vi "Get Coincident Pairs.vi"(4 "interp. method":enum16{"nearest", "linear"}(ring)=enum."linear", 6 "Array 2 Time (s) offset (Default 0)":dbl, 8 "Index2":i32, 9 "Index1":i32, 10 "Cluster 2":T2={"Colour"=0, "Inst type"=enum."Pitot-static tube", "Inst name"="Manometer voltage", "Symbol"="U", "Code name"="", "Extra Info"="U", "Inst Array"=enum."PWA", "U"=0.0, "u^2"=0.0, "u^3"=0.0, "u^4"=0.0, "Skew_u"=0.0, "Kurt_u"=0.0, "Sd Error in Mean"=0.0, "% u'/U"=0.0, "X"=0.0, "Y"=0.0, "Z"=0.0, "Timescale integral Estimate"=0.0, "Sd Error in Variance"=0.0, "Calib File"=path "", "Calib Constants"=[], "Output Position"=FALSE, "Stats"=enum."None", "Av Sampling Rate"=0.0, "Av No of Samples"=0.0, "Total Meas Time (s)"=0.0, "OrigChName"="", "Max value"=0.0, "Min value"=0.0, "Req Sample Rate Hz"=0.0, "Sync Delay Time (s)"=0.0, "Ch No"=0, "Device"="", "Use Latest Calib"=FALSE, "Port"="", "Metadata Ch Names"=[], "Metadata Ch Values"=[], "Label"="", "chState"=enum."Solo", "Point Drift"=0.0, "inputConfig"=""} {"Kurt_u" format="%_3g"; "u^4" format="%_3g"; "u^3" format="%_3g"; "Sd Error in Variance" format="%_3g"; "u^2" format="%_3g"; "Sd Error in Mean" format="%_3g"; "U" format="%_3g"; "Sync Delay Time (s)" format="%.4f"; "Total Meas Time (s)" format="%_5g"; "Skew_u" format="%_3g"; "% u'/U" format="%_3g"}, 11 "Cluster 1":T2={"Colour"=0, "Inst type"=enum."Pitot-static tube", "Inst name"="Manometer voltage", "Symbol"="U", "Code name"="", "Extra Info"="U", "Inst Array"=enum."PWA", "U"=0.0, "u^2"=0.0, "u^3"=0.0, "u^4"=0.0, "Skew_u"=0.0, "Kurt_u"=0.0, "Sd Error in Mean"=0.0, "% u'/U"=0.0, "X"=0.0, "Y"=0.0, "Z"=0.0, "Timescale integral Estimate"=0.0, "Sd Error in Variance"=0.0, "Calib File"=path "", "Calib Constants"=[], "Output Position"=FALSE, "Stats"=enum."None", "Av Sampling Rate"=0.0, "Av No of Samples"=0.0, "Total Meas Time (s)"=0.0, "OrigChName"="", "Max value"=0.0, "Min value"=0.0, "Req Sample Rate Hz"=0.0, "Sync Delay Time (s)"=0.0, "Ch No"=0, "Device"="", "Use Latest Calib"=FALSE, "Port"="", "Metadata Ch Names"=[], "Metadata Ch Values"=[], "Label"="", "chState"=enum."Solo", "Point Drift"=0.0, "inputConfig"=""} {"Kurt_u" format="%_3g"; "u^4" format="%_3g"; "u^3" format="%_3g"; "Sd Error in Variance" format="%_3g"; "u^2" format="%_3g"; "Sd Error in Mean" format="%_3g"; "U" format="%_3g"; "Sync Delay Time (s)" format="%.4f"; "Total Meas Time (s)" format="%_5g"; "Skew_u" format="%_3g"; "% u'/U" format="%_3g"}) -> (0 "Pairs":cluster{"Cluster":T1, "Cluster":T1, dbl}, 3 "Need to Update":bool)   [LabVIEW 2022 SP3]
uses:
  Globals/Meas_global.vi
  Controls/Inst_type.ctl
  Controls/Instrument_Array.ctl
  Controls/Analysis_info_cluster.ctl
  Controls/Resample mode.ctl
  Controls/channelState.ctl
panel:
  out "Array":cluster{"Index1":i32, "Index2":i32}[](array[cluster])
  out "Time Window (ms)":dbl
  out "Frame":string
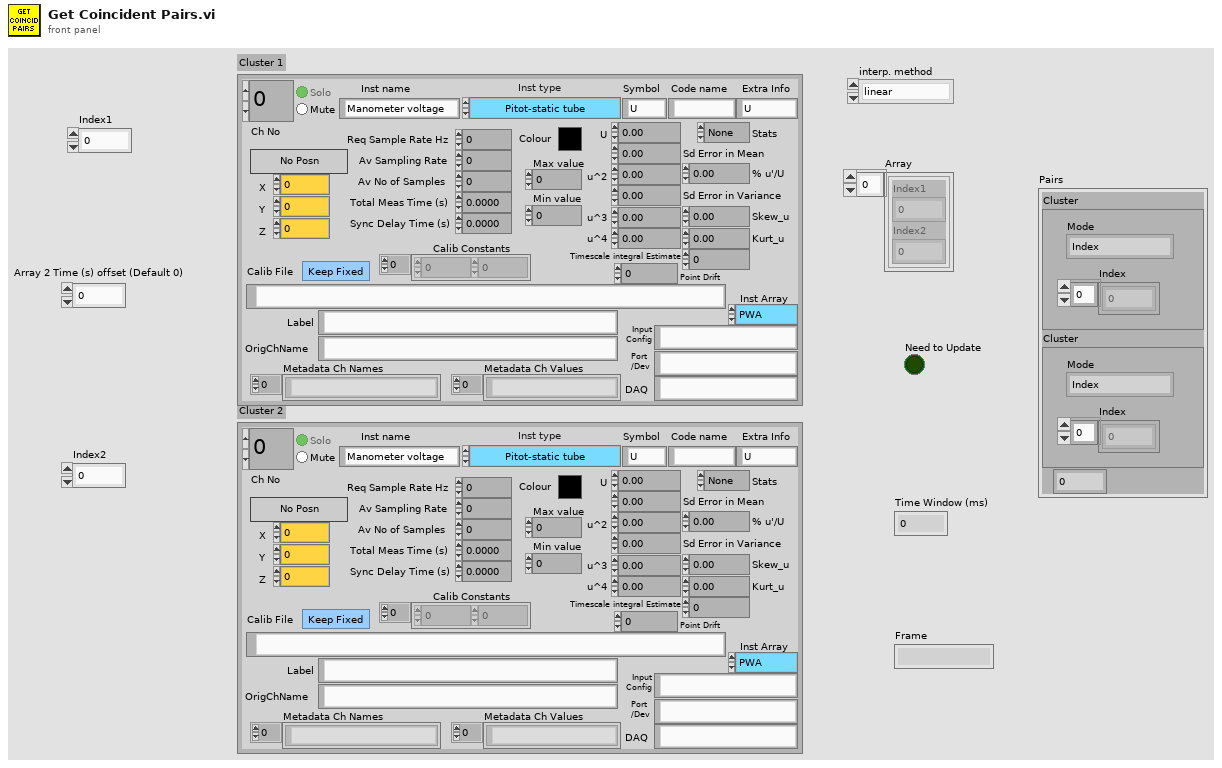
[diagram p1: front panel]
types:
  T1 = typedef "Resample mode.ctl" = cluster{"Mode":enum16{"Index", "Interpolate"}, "Index":dbl[]}
  T2 = typedef "Analysis_info_cluster.ctl" = cluster{"Colour":u32, "Inst type":T3, "Inst name":string, "Symbol":string, "Code name":string, "Extra Info":string, "Inst Array":T4, "U":dbl, "u^2":dbl, "u^3":dbl, "u^4":dbl, "Skew_u":dbl, "Kurt_u":dbl, "Sd Error in Mean":dbl, "% u'/U":dbl, "X":dbl, "Y":dbl, "Z":dbl, "Timescale integral Estimate":dbl, "Sd Error in Variance":dbl, "Calib File":path, "Calib Constants":dbl[], "Output Position":bool, "Stats":enum16{"None", "Basic", "Full"}, "Av Sampling Rate":dbl, "Av No of Samples":dbl, "Total Meas Time (s)":dbl, "OrigChName":string, "Max value":dbl, "Min value":dbl, "Req Sample Rate Hz":dbl, "Sync Delay Time (s)":dbl, "Ch No":i16, "Device":string, "Use Latest Calib":bool, "Port":string, "Metadata Ch Names":string[], "Metadata Ch Values":string[], "Label":string, "chState":T5, "Point Drift":dbl, "inputConfig":string}
  T3 = typedef "Inst_type.ctl" = enum16{"Raw voltage", "Raw with zero offsetting", "Propeller anemometer", "Pressure Transducer", "Pitot-static tube", "Hot wire", "Cross wire 1", "Cross wire 2", "Generic Linear", "Generic Polynomial", "Generic BackPoly", "Fast FID", "Thermocouple", "Cold wire", "Pulsed Wire", "LDA Vel", "LDA Tran time", "LDA Arr time", "Microphone"}
  T4 = typedef "Instrument_Array.ctl" = enum16{"PWA", "LDA", "Analogue"}
  T5 = typedef "channelState.ctl" = enum32{"No Selection", "Solo", "Mute"}
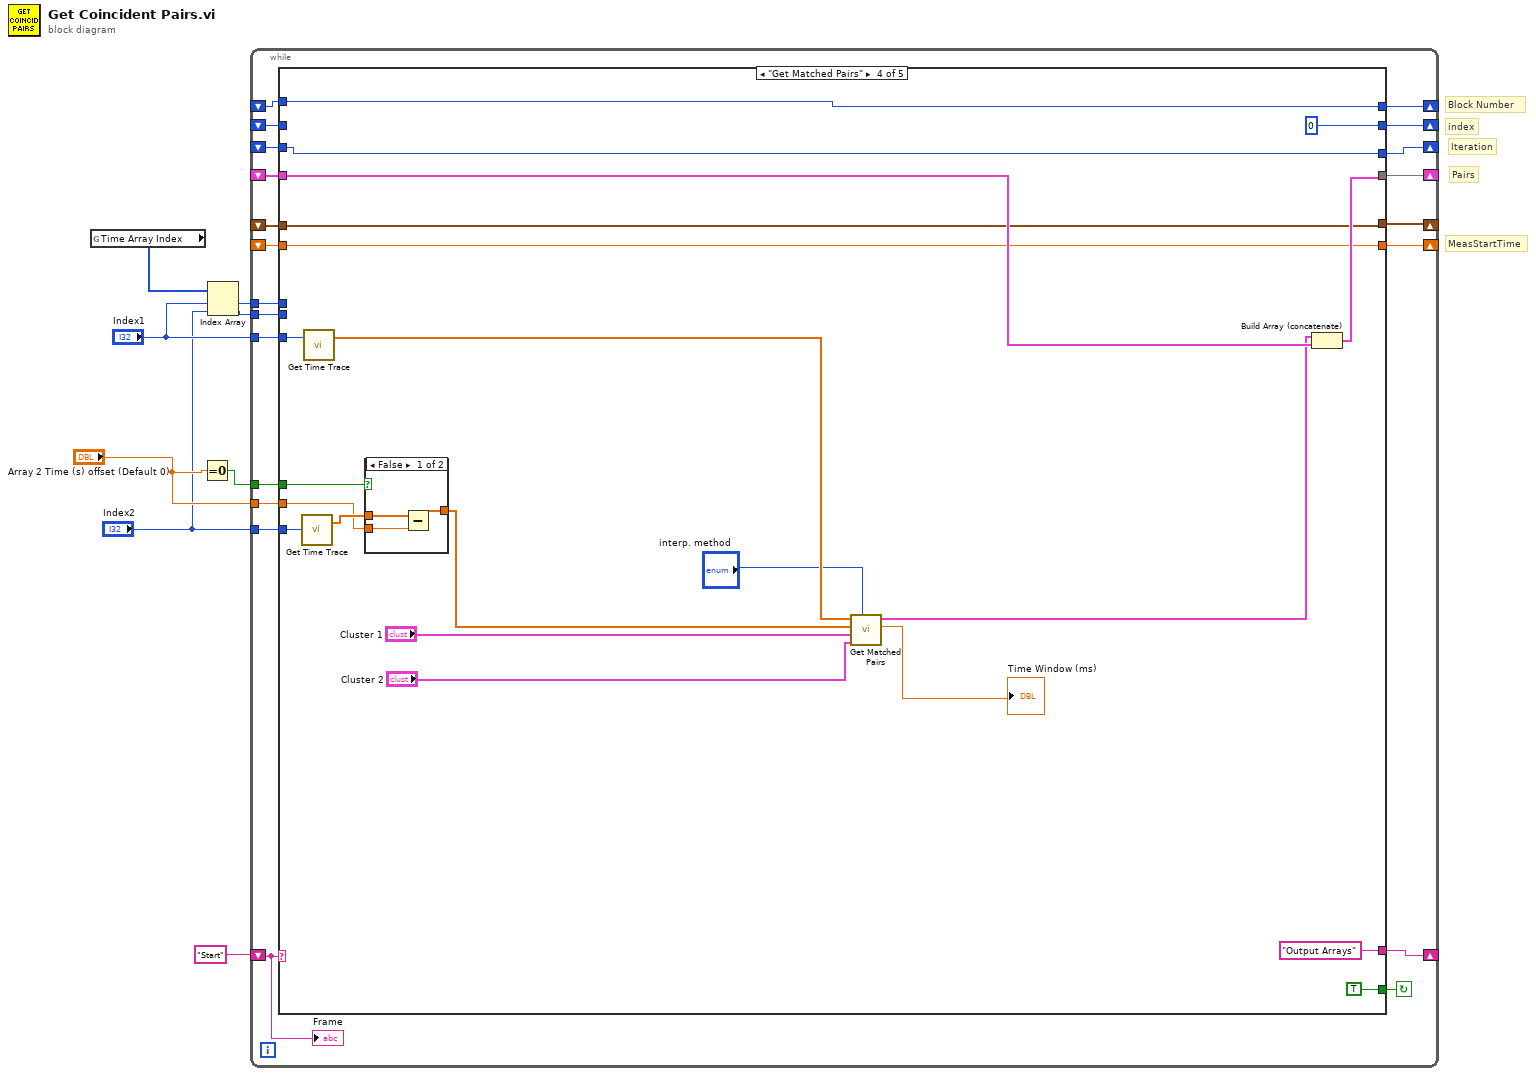
[diagram p0: block diagram]
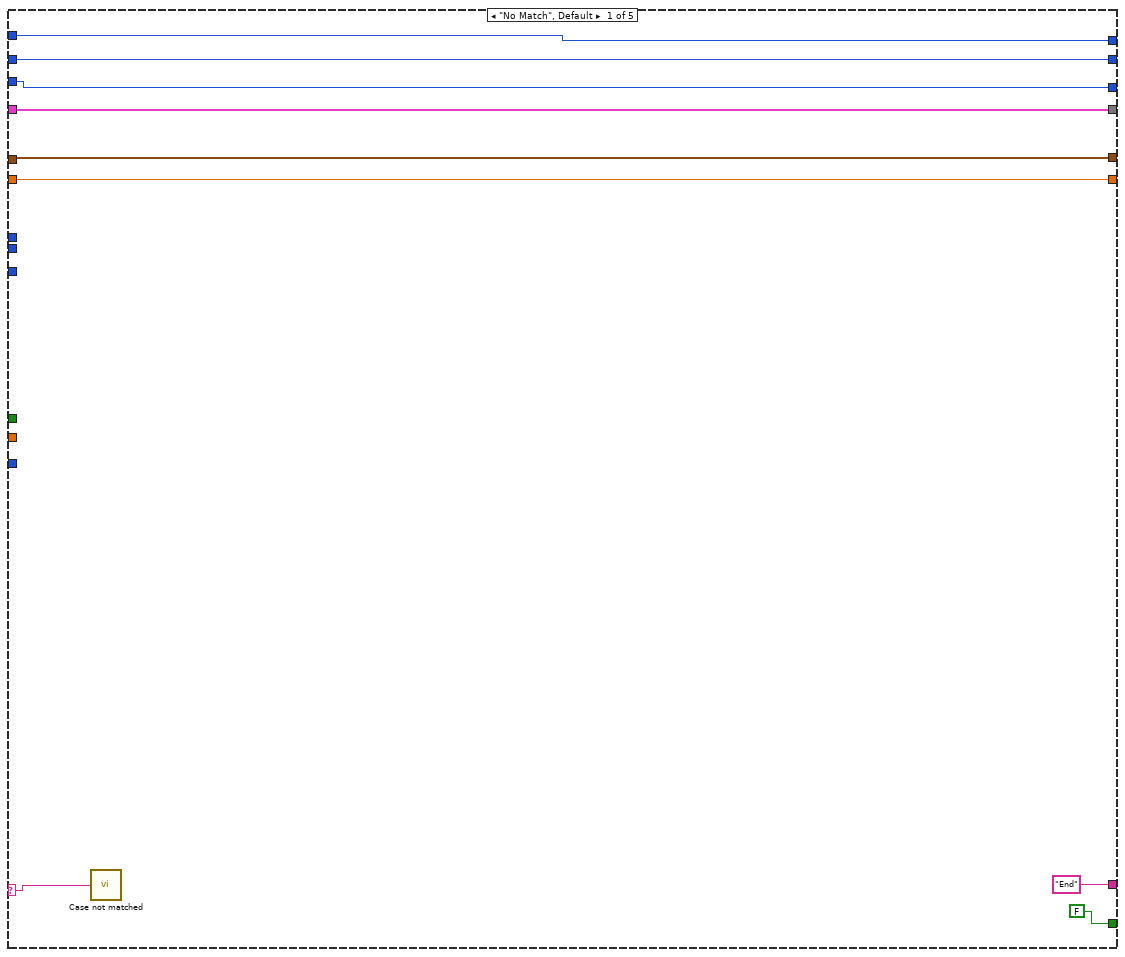
[diagram p2: hidden frame]
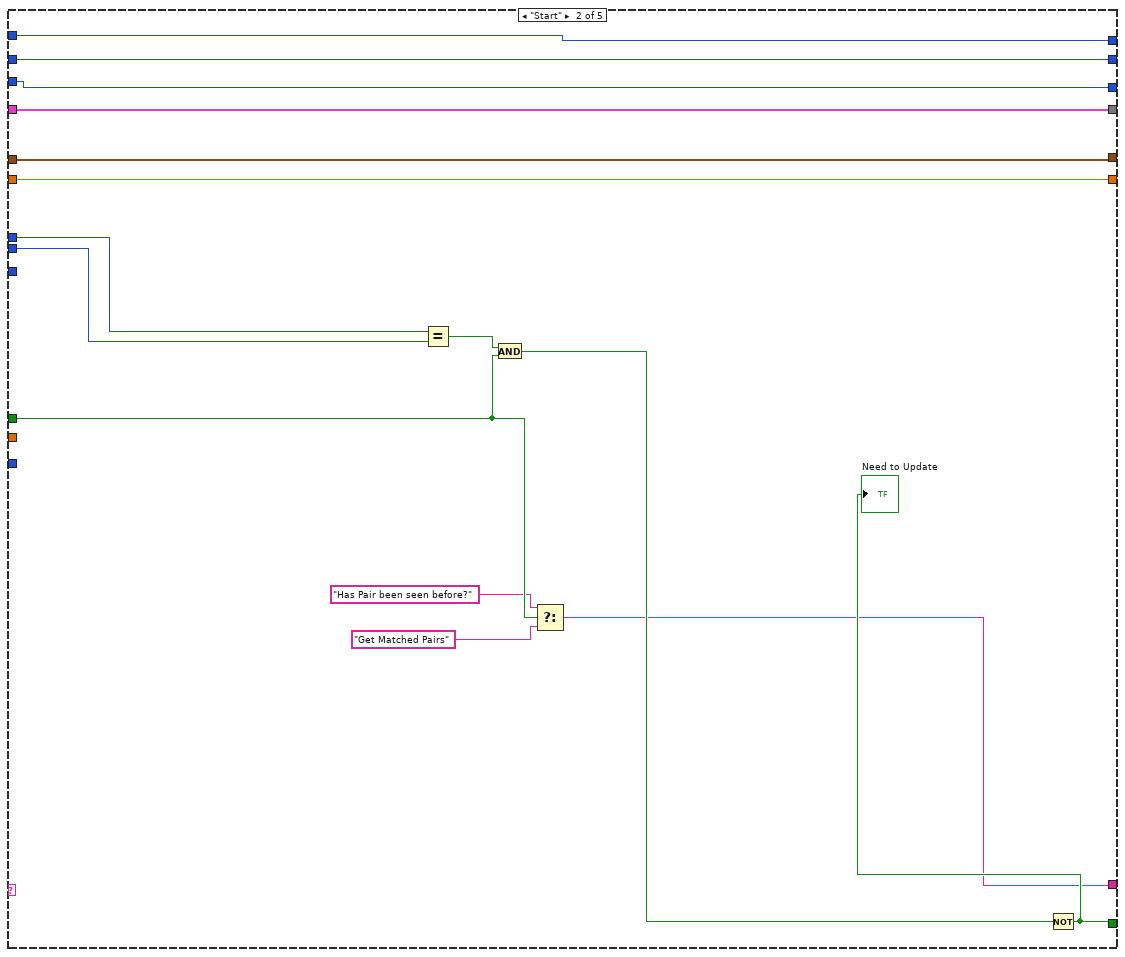
[diagram p3: hidden frame]
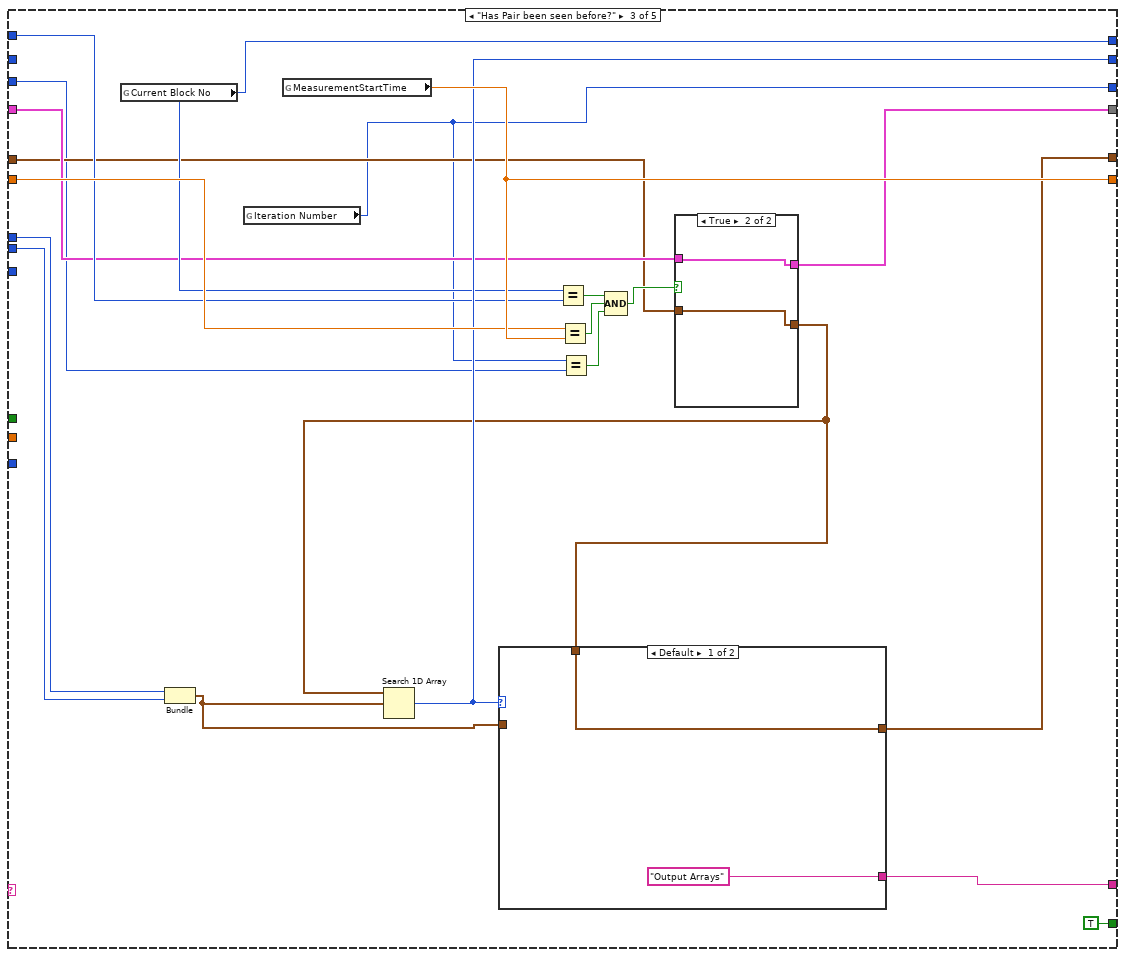
[diagram p4: hidden frame]
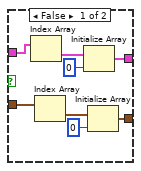
[diagram p5: hidden frame]
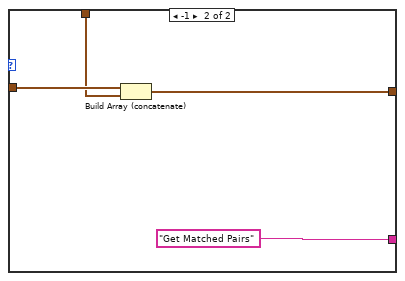
[diagram p6: hidden frame]
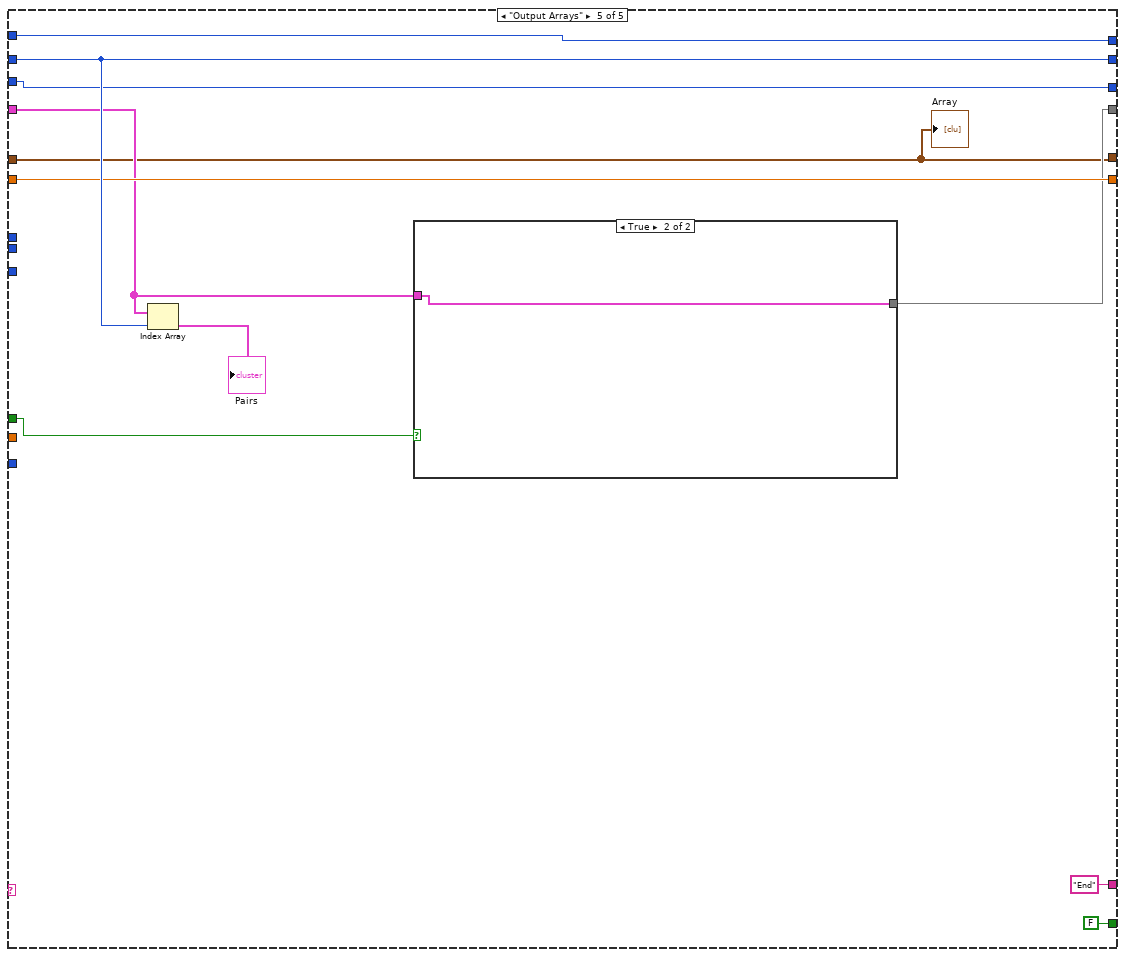
[diagram p8: hidden frame]
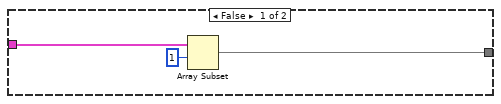
[diagram p9: hidden frame]
diagram:
  # "MeasStartTime"
  # "Pairs"
  # "Iteration"
  # "index"
  # "Block Number"
  n1 = global read "Meas_global.vi" "Time Array Index"() -> (w5:i32[])
  n2 = Equal To 0?(x="Array 2 Time (s) offset (Default 0)") -> (x = 0?=w7:bool)
  n3 = Index Array(array=w5, index #1="Index1", index #2="Index2") -> (element #1=w2:i32, element #2=w1:i32)
  n4 = while {
    shift-right: [w27] -> _
    shift-left: "Start" -> [w29]
    shift-right: [w26] -> _
    shift-left: _ -> [w25]
    tunnel: "Index1" -> [w24]
    tunnel: "Index2" -> [w23]
    shift-right: [w20] -> _
    shift-left: _ -> [w19]
    shift-right: [w22] -> _
    shift-left: _ -> [w21]
    shift-right: [w18] -> _
    shift-left: _ -> [w17]
    shift-right: [w16] -> _
    shift-left: _ -> [w15]
    shift-right: [w14] -> _
    shift-left: _ -> [w13]
    tunnel: "Array 2 Time (s) offset (Default 0)" -> [w11]
    tunnel: w7 -> [w12]
    tunnel: w2 -> [w10]
    tunnel: w1 -> [w9]
    stop <- w28 continue-if-true
    n5 = case shown="\"Get Matched Pairs\"" w29 {
      selector: w29 -> [w35 _ _ _ _]
      tunnel: [FALSE w47 TRUE TRUE FALSE] -> w28
      tunnel: ["End" w42 w65 "Output Arrays" "End" ("t")] -> w27
      tunnel: [w36 w51 w61 w108 w118] -> w26
      tunnel: w25 -> [w36 w51 w63 w109 w119]
      tunnel: w24 -> [_ _ _ w106 _]
      tunnel: w23 -> [_ _ _ w105 _]
      tunnel: [w31 w49 w74 w101 w122] -> w22
      tunnel: w21 -> [w31 w49 w73 w101 w122]
      tunnel: [w32 w50 w72 w102 w116] -> w20
      tunnel: w19 -> [w32 w50 w60 w102 w116]
      tunnel: [w33 w52 w70 0 w126] -> w18
      tunnel: w17 -> [w33 w52 _ _ w126]
      tunnel: [w34 w53 w69 w103 w123] -> w16
      tunnel: w15 -> [w34 w53 w68 w103 w123]
      tunnel: [w30 w48 w57 w99 w121] -> w14
      tunnel: w13 -> [w30 w48 w56 w99 w121]
      tunnel: w12 -> [_ w44 _ w96 w120]
      tunnel: w11 -> [_ _ _ w95 _]
      tunnel: w10 -> [_ w40 w55 _ _]
      tunnel: w9 -> [_ w39 w54 _ _]
      frame "No Match", Default {
        n6 = call "Case not matched.vi"("Case Name not Matched"=w35) -> ()
      }
      frame "Start" {
        n7 = Equal?(x=w40, y=w39) -> (x = y?=w46:bool)
        n8 = And(x=w46, y=w44) -> (x .and. y?=w45:bool)
        n9 = Select(t="Has Pair been seen before?", s=w44, f="Get Matched Pairs" ("t")) -> (s? t:f=w42:string)
        n10 = Not(x=w45) -> (.not. x?=w47:bool)
        "Need to Update" <- w47
      }
      frame "Has Pair been seen before?" {
        n11 = global read "Meas_global.vi" "Current Block No"() -> (w69:i32)
        n12 = Bundle("Numeric"=w55, "Numeric"=w54) -> (w71:cluster{"Numeric":i32, "Numeric":i32})  [unwired: 1 in]
        n13 = global read "Meas_global.vi" "Iteration Number"() -> (w57:i32)
        n14 = global read "Meas_global.vi" "MeasurementStartTime"() -> (w74:dbl)
        n15 = Equal?(x=w69, y=w68) -> (x = y?=w67:bool)
        n16 = Equal?(x=w73, y=w74) -> (x = y?=w66:bool)
        n17 = Equal?(x=w57, y=w56) -> (x = y?=w58:bool)
        n18 = Compound Arithmetic op=AND(w67, w66, w58) -> (w62:bool)
        n19 = case shown="True" w62 {
          tunnel: w63 -> [w82 w84]
          tunnel: [w79 w84] -> w61
          tunnel: w60 -> [w76 w83]
          tunnel: [w75 w83] -> w59
          frame False {
            n20 = Index Array(array=w82) -> (element=w81:cluster{"Cluster":T1, "Cluster":T1, dbl})  [unwired: 1 in]
            n21 = Index Array(array=w76) -> (element=w77:cluster{"Numeric":i32, "Numeric":i32})  [unwired: 1 in]
            n22 = Initialize Array(w81, 0 ("dimension size")) -> (w79:cluster{"Cluster":T1, "Cluster":T1, dbl}[])
            n23 = Initialize Array(w77, 0 ("dimension size")) -> (w75:cluster{"Numeric":i32, "Numeric":i32}[])
          }
          frame True {
          }
        }
        n24 = Search 1D Array(1D array=w59, element=w71) -> (index of element=w70:i32)  [unwired: 1 in]
        n25 = case shown="Default" w70 {
          tunnel: w71 -> [_ w89]
          tunnel: [w86 w90] -> w72
          tunnel: w59 -> [w86 w88]
          tunnel: ["Output Arrays" ("t") "Get Matched Pairs" ("t")] -> w65
          frame Default {
          }
          frame -1 {
            n26 = Build Array (concatenate)(w89, w88) -> (w90:cluster{"Numeric":i32, "Numeric":i32}[])
          }
        }
      }
      frame "Get Matched Pairs" {
        n27 = call "Get Time Trace.vi"("Channel Index"=w105) -> ("Time (s)"=w98:dbl[])  [unwired: 1 out]
        n28 = call "Get Time Trace.vi"("Channel Index"=w106) -> ("Time (s)"=w104:dbl[])  [unwired: 1 out]
        n29 = case shown="False" w96 {
          tunnel: w95 -> [w114 _]
          tunnel: w98 -> [w113 w115]
          tunnel: [w112 w115] -> w97
          frame False {
            n30 = Subtract(x=w113, y=w114) -> (x-y=w112:dbl[])
          }
          frame True {
          }
        }
        n31 = call "Get Matched Pairs.vi"("interp. method"="interp. method", "Cluster 2"="Cluster 2", "Cluster 1"="Cluster 1", "Time (s) 2"=w97, "Time (s) 1"=w104) -> ("Time Window (ms)"=→"Time Window (ms)":dbl, "Cluster out"=w93:cluster{"Cluster":T1, "Cluster":T1, dbl})  [unwired: 5 in]
        n32 = Build Array (concatenate)(w93, w109) -> (w108:cluster{"Cluster":T1, "Cluster":T1, dbl}[])
      }
      frame "Output Arrays" {
        n33 = Index Array(array=w119, index=w126) -> (element=→"Pairs":cluster{"Cluster":T1, "Cluster":T1, dbl})
        n34 = case shown="True" w120 {
          tunnel: w119 -> [w129 w130]
          tunnel: [w127 w130] -> w118
          frame False {
            n35 = Array Subset(array=w129, index=1) -> (w127:cluster{"Cluster":T1, "Cluster":T1, dbl}[])  [unwired: 1 in]
          }
          frame True {
          }
        }
        "Array" <- w116
      }
    }
    "Frame" <- w29
  }
